vi "SLSC_Out.vi"(6 "SLSC Dynamic Outputs":T1[](array[typedef]), 8 "error in":errorcluster, 9 "Values":dbl[](array[numeric]), 10 "session in":refnum<k21>, 11 "SLSC Module Name":refnum<k21>) -> (0 "error out":errorcluster, 1 "LoopRate(ms)":u32=50, 2 "session out":refnum<k21>, 3 "SLSC Module Name":refnum<k21>)   [LabVIEW 2020]
uses:
  <vilib>/SLSC/SLSC.lvlib
  <vilib>/SLSC/Set Generic Property (String).vi
  <vilib>/SLSC/Set Generic Property (U64).vi
  <vilib>/SLSC/Set Generic Property (I64).vi
  <vilib>/SLSC/Set Generic Property (I32).vi
  <vilib>/SLSC/Set Generic Property (DBL).vi
  <vilib>/SLSC/Set Generic Property (Bool).vi
  <vilib>/SLSC/Set Generic Property (U32).vi
  <vilib>/SLSC/Commit Properties for Devices.vi
  SLSC Dynamic Channel.ctl
  SLSC Datatype.ctl
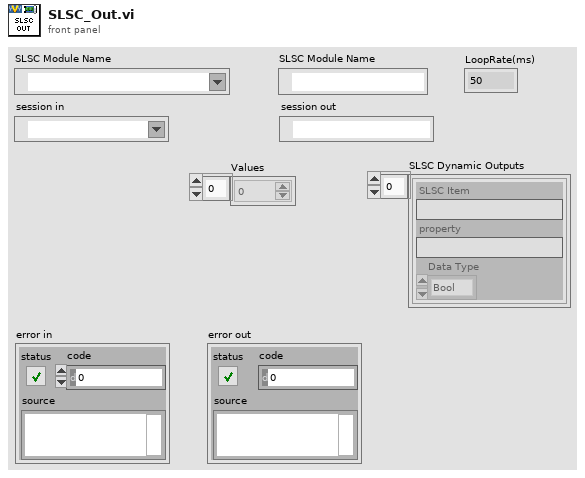
[diagram p1: front panel]
types:
  T1 = typedef "SLSC CD Engine.lvlib/SLSC Dynamic Channel.ctl" = cluster{"SLSC Item":string, "property":string, "Data Type":T2}
  T2 = typedef "SLSC CD Engine.lvlib/SLSC Datatype.ctl" = enum16{"Bool", "Double", "I32", "I64", "String", "U32", "U64"}
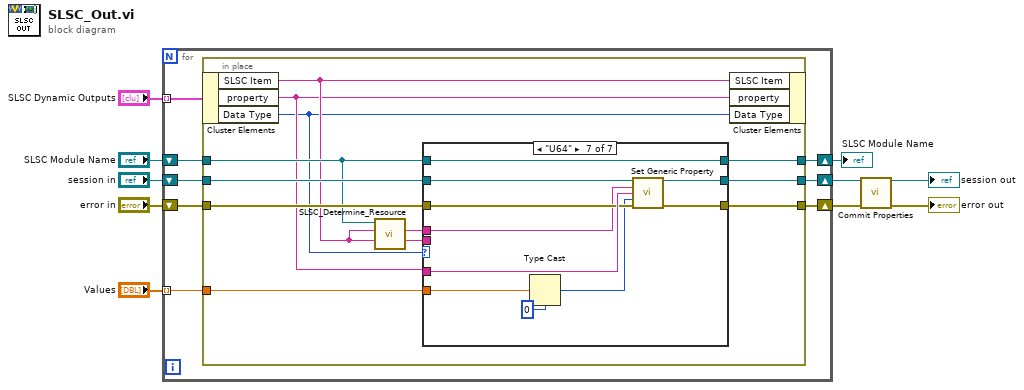
[diagram p0: block diagram]
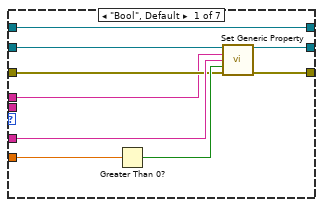
[diagram p2: hidden frame]
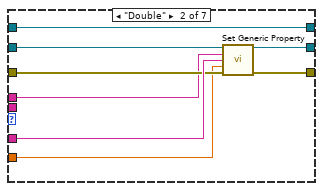
[diagram p3: hidden frame]
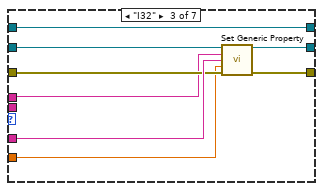
[diagram p4: hidden frame]
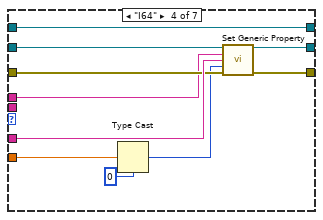
[diagram p5: hidden frame]
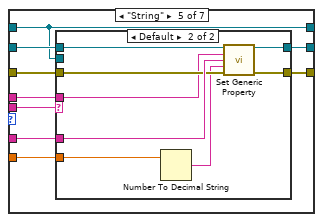
[diagram p6: hidden frame]
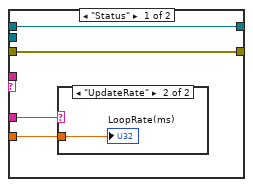
[diagram p7: hidden frame]
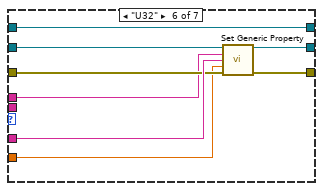
[diagram p9: hidden frame]
diagram:
  n1 = for {
    tunnel: "Values" -> [w18] mode=indexing
    tunnel: "SLSC Dynamic Outputs" -> [w11] mode=indexing
    shift-right: [w16] -> w2
    shift-left: "session in" -> [w17]
    shift-right: [w15] -> w5
    shift-left: "SLSC Module Name" -> [w12]
    shift-right: [w13] -> w4
    shift-left: "error in" -> [w14]
    n2 = in-place {
      in-place-border: w18 -> [w29]
      in-place-border: w17 -> [w28]
      in-place-border: [w27] -> w16
      in-place-border: [w26] -> w15
      in-place-border: w14 -> [w25]
      in-place-border: [w24] -> w13
      in-place-border: w12 -> [w23]
      n3 = in-place-cluster #1(w11) -> ("SLSC Item"=w21:string, "property"=w20:string, "Data Type"=w19:T2)
      n4 = call "SLSC_Determine_Resource.vi"("SLSC Item"=w21, "SLSC Module Name"=w23) -> ("Resource"=w22:string)  [unwired: 9 in]
      n5 = case shown="\"U64\"" w19 {
        tunnel: w29 -> [w38 w40 w48 w58 w68 w88 w97]
        tunnel: w28 -> [w36 w46 w54 w64 w73 w94 w104]
        tunnel: [w35 w45 w53 w63 w72 w93 w103] -> w27
        tunnel: w20 -> [w34 w44 w52 w62 w71 w92 w102]
        tunnel: w23 -> [w33 w43 w51 w61 w67 w91 w101]
        tunnel: [w33 w43 w51 w61 w67 w91 w101] -> w26
        tunnel: w25 -> [w32 w42 w50 w60 w70 w90 w100]
        tunnel: [w31 w41 w49 w59 w69 w89 w99] -> w24
        tunnel: w22 -> [w30 w39 w47 w55 w65 w87 w95]
        tunnel: w21 -> [_ _ _ _ w66 _ _]
        frame "Bool", Default {
          n6 = Greater Than 0?(x=w38) -> (x > 0?=w37:bool)
          n7 = call-poly <vilib>:"Set Generic Property.vi"("session in"=w36, "resources"=w30, "property"=w34, "property value"=w37, "error in (no error)"=w32) -> ("session out"=w35:refnum<k21>, "error out"=w31:errorcluster)  [unwired: 9 in]
        }
        frame "Double" {
          n8 = call-poly <vilib>:"Set Generic Property.vi"("session in"=w46, "resources"=w39, "property"=w44, "property value"=w40, "error in (no error)"=w42) -> ("session out"=w45:refnum<k21>, "error out"=w41:errorcluster)  [unwired: 9 in]
        }
        frame "I32" {
          n9 = call-poly <vilib>:"Set Generic Property.vi"("session in"=w54, "resources"=w47, "property"=w52, "property value"=w48, "error in (no error)"=w50) -> ("session out"=w53:refnum<k21>, "error out"=w49:errorcluster)  [unwired: 9 in]
        }
        frame "I64" {
          n10 = Type Cast(type=i64 0 ("property value"), x=w58) -> (*(type *) &x=w56:i64)
          n11 = call-poly <vilib>:"Set Generic Property.vi"("session in"=w64, "resources"=w55, "property"=w62, "property value"=w56, "error in (no error)"=w60) -> ("session out"=w63:refnum<k21>, "error out"=w59:errorcluster)  [unwired: 9 in]
        }
        frame "String" {
          n12 = case shown="Default" w66 {
            tunnel: w73 -> [w76 w86]
            tunnel: [w76 w85] -> w72
            tunnel: w71 -> [w74 w84]
            tunnel: w67 -> [_ _]
            tunnel: w70 -> [w77 w83]
            tunnel: [w77 w82] -> w69
            tunnel: w68 -> [w75 w81]
            tunnel: w65 -> [_ w79]
            frame "Status" {
              n13 = case shown="\"UpdateRate\"" w74 {
                tunnel: w75 -> [_ w78]
                frame Default {
                }
                frame "UpdateRate" {
                  "LoopRate(ms)" <- w78
                }
              }
            }
            frame Default {
              n14 = Number To Decimal String(number=w81) -> (decimal integer string=w80:string)  [unwired: 1 in]
              n15 = call-poly <vilib>:"Set Generic Property.vi"("session in"=w86, "resources"=w79, "property"=w84, "property value"=w80, "error in (no error)"=w83) -> ("session out"=w85:refnum<k21>, "error out"=w82:errorcluster)  [unwired: 9 in]
            }
          }
        }
        frame "U32" {
          n16 = call-poly <vilib>:"Set Generic Property.vi"("session in"=w94, "resources"=w87, "property"=w92, "property value"=w88, "error in (no error)"=w90) -> ("session out"=w93:refnum<k21>, "error out"=w89:errorcluster)  [unwired: 9 in]
        }
        frame "U64" {
          n17 = Type Cast(type=u64 0 ("property value"), x=w97) -> (*(type *) &x=w96:u64)
          n18 = call-poly <vilib>:"Set Generic Property.vi"("session in"=w104, "resources"=w95, "property"=w102, "property value"=w96, "error in (no error)"=w100) -> ("session out"=w103:refnum<k21>, "error out"=w99:errorcluster)  [unwired: 9 in]
        }
      }
      n19 = in-place-cluster #1("SLSC Item"=w21, "property"=w20, "Data Type"=w19) -> ()  [unwired: 1 out]
    }
  }
  "SLSC Module Name" <- w5
  n20 = call-poly <vilib>:"Commit Properties.vi"("session in"=w2, "error in (no error)"=w4) -> ("session out"=→"session out":refnum<k21>, "error out"=→"error out":errorcluster)  [unwired: 12 in]
